vi "test2.vi"() -> ()   [LabVIEW 2023]
uses:
  Devices/Rigol DS1054/Rigol DS1054.lvclass
  D:/git/HAL/Scope Base/Scope Base.lvclass
  Camera Base/Acquisition Stats.ctl
  Devices/PXIe-5172 Simulated/PXIe-5172 Simulated.lvclass
  Devices/PXIe-5172 Simulated/configurations/Fetch 10kHz_class/Continuous Waveform Acq CFG.lvclass
  D:/git/HAL/Configuration Base/Configuration Base.lvclass
  Devices/Rigol DS1054/Configurations/Acquire Continuous Waveform/Continuous Waveform Acq CFG.lvclass
  Configuration Base/Configuration Base.lvclass
  D:/git/HAL/Interfaces/IConfigure/IConfigure.lvclass
  Scope Base/Scope Base.lvclass
  Devices/Flir A700/Flir A700.lvclass
  Camera Imaqdx/Configuration/Camera Imaqdx CFG.lvclass
  Camera Base/Camera Base.lvclass
  D:/git/HAL/Camera Base/Camera Base.lvclass
panel:
  out "Acquisition Stats":T1
  out "Image":T2(plugin-control)
  out "error out cams":errorcluster
  out "error out scopes":errorcluster
  out "Error Out":errorcluster
  in  "RIGOL DS1054.lvlib:Rigol DS1054.lvclass":refnum<class "Rigol DS1054.lvclass">
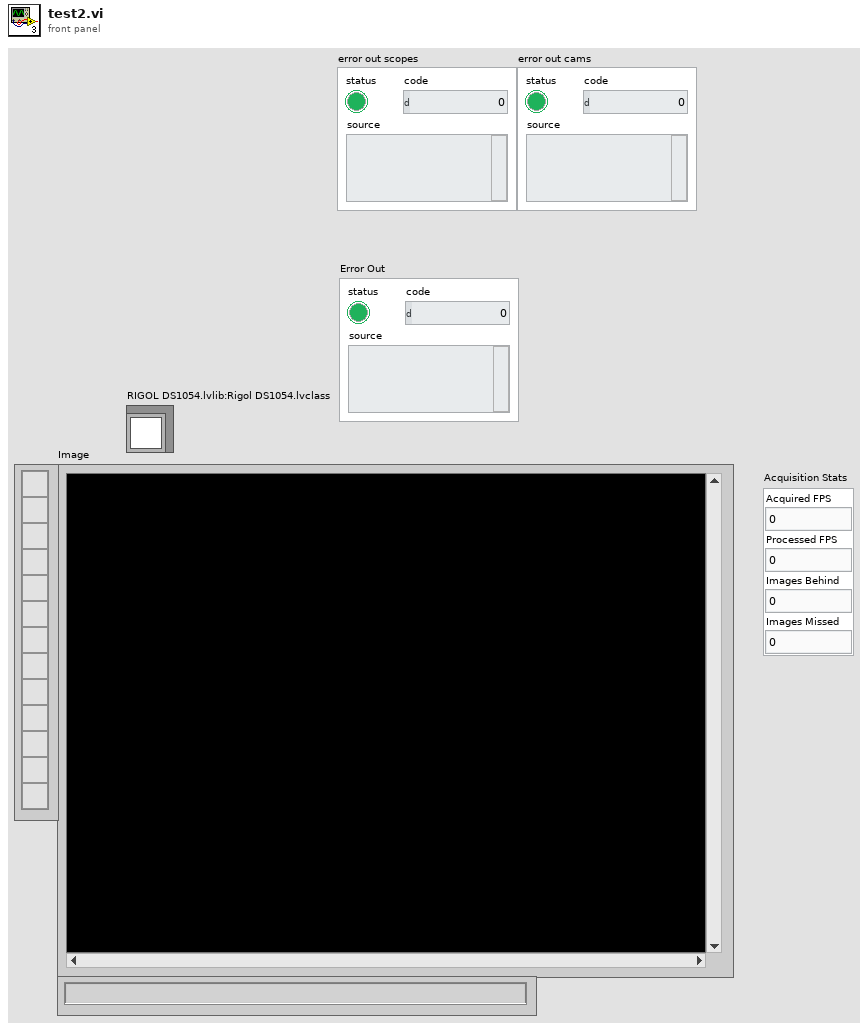
[diagram p1: front panel]
types:
  T1 = typedef "HAL.lvlib/Camera Base.lvclass/Acquisition Stats.ctl" = cluster{"Acquired FPS":dbl, "Processed FPS":dbl, "Images Behind":u32, "Images Missed":u32}
  T2 = typedef "IMAQ Image.ctl" = refnum<image>
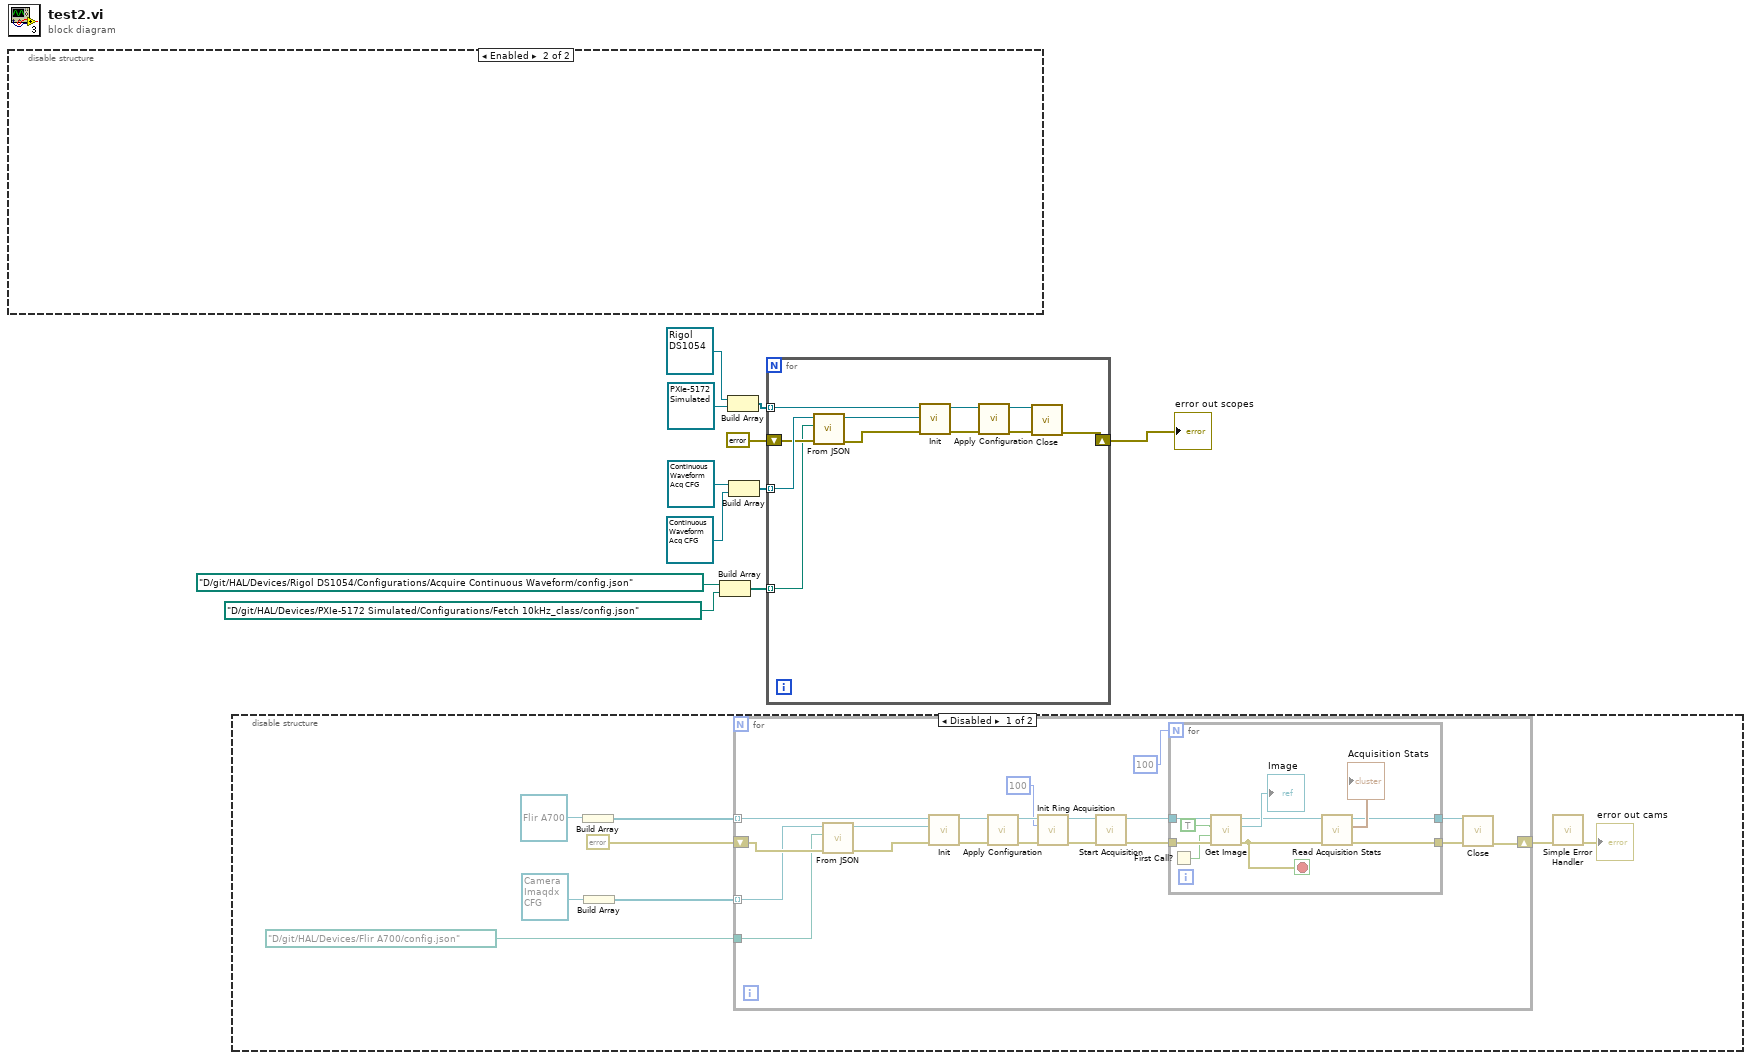
[diagram p0: block diagram]
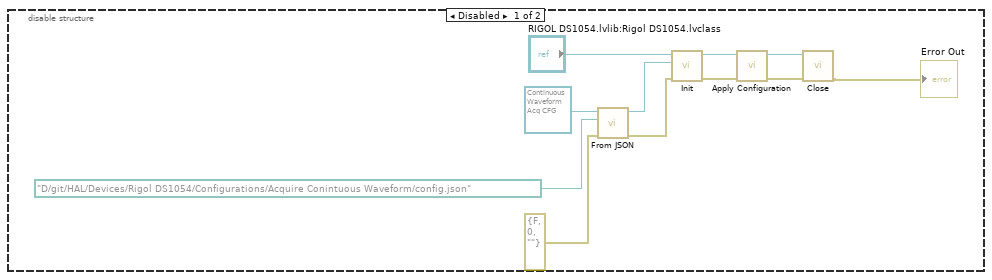
[diagram p3: hidden frame]
diagram:
  n1 = disable-structure shown="Enabled" {
    frame Disabled {
      n2 = call-dynamic "From JSON.vi"("error in (no error)"=errorcluster {"status"=FALSE, "code"=0, "source"=""} ("Error In"), "JSON Config"=path "D:/git/HAL/Devices/Rigol DS1054/Configurations/Acquire Conintuous Waveform/config.json" ("File Path"), "Camera Config in"=refnum<class "Continuous Waveform Acq CFG.lvclass"> refnum ("RIGOL DS1054.lvlib:Acquire Continuous Waveform CFG.lvclass")) -> ("error out"=w12:errorcluster, "Camera Config out"=w21:refnum<class "Continuous Waveform Acq CFG.lvclass">)  [unwired: 7 in]
      n3 = call-dynamic "Init.vi"("Error In"=w12, "IConfigure"=w21, "object in"="RIGOL DS1054.lvlib:Rigol DS1054.lvclass") -> ("Error Out"=w17:errorcluster, "object out"=w18:refnum<class "Rigol DS1054.lvclass">)  [unwired: 7 in]
      n4 = call "Apply Configuration.vi"("error in (no error)"=w17, "Rigol DS1054 in"=w18) -> ("error out"=w15:errorcluster, "Rigol DS1054 out"=w16:refnum<class "Rigol DS1054.lvclass">)  [unwired: 8 in]
      n5 = call-dynamic "Close.vi"("Error In"=w15, "object in"=w16) -> ("Error Out"=→"Error Out":errorcluster)  [unwired: 8 in, 1 out]
    }
    frame Enabled {
    }
  }
  n6 = disable-structure shown="Disabled" {
    frame Disabled {
      n7 = Build Array(refnum<class "Flir A700.lvclass"> refnum ("FLIR A700.lvlib:Flir A700.lvclass")) -> (w27:refnum<class "Flir A700.lvclass">[])
      n8 = Build Array(refnum<class "Camera Imaqdx CFG.lvclass"> refnum ("HAL.lvlib:Camera Imaqdx CFG.lvclass")) -> (w28:refnum<class "Camera Imaqdx CFG.lvclass">[])
      n9 = for {
        tunnel: w27 -> [w49] mode=indexing
        tunnel: w28 -> [w43] mode=indexing
        shift-right: [w45] -> w30
        shift-left: errorcluster {"status"=FALSE, "code"=0, "source"=""} ("error constant") -> [w48]
        tunnel: path "D:/git/HAL/Devices/Flir A700/config.json" ("JSON Config") -> [w41]
        n10 = call-dynamic "From JSON.vi"("error in"=w48, "JSON Config"=w41, "Camera Config Imaqdx in"=w43) -> ("error out"=w44:errorcluster, "Camera Config Imaqdx out"=w42:refnum<class "Camera Imaqdx CFG.lvclass">)  [unwired: 7 in]
        n11 = call-dynamic "Init.vi"("error in (no error)"=w44, "IConfigure"=w42, "Flir A700 in"=w49) -> ("error out"=w47:errorcluster, "Flir A700 out"=w46:refnum<class "Flir A700.lvclass">)  [unwired: 7 in]
        n12 = call-dynamic "Apply Configuration.vi"("error in (no error)"=w47, "Camera Base in"=w46) -> ("error out"=w39:errorcluster, "Camera Base out"=w38:refnum<class "Flir A700.lvclass">)  [unwired: 8 in]
        n13 = call-dynamic "Init Ring Acquisition.vi"("error in (no error)"=w39, "Ring Buffer Size"=u32 100, "Camera Imaqdx in"=w38) -> ("error out"=w36:errorcluster, "Camera Imaqdx out"=w35:refnum<class "Flir A700.lvclass">)  [unwired: 7 in]
        n14 = call-dynamic "Start Acquisition.vi"("error in"=w36, "Camera Imaqdx in"=w35) -> ("error out"=w33:errorcluster, "Camera Imaqdx out"=w34:refnum<class "Flir A700.lvclass">)  [unwired: 8 in]
        n15 = for {
          N: 100 -> [_]
          tunnel: w34 -> [w58]
          tunnel: w33 -> [w59]
          tunnel: [w51] -> w32
          tunnel: [w50] -> w31
          stop <- w54 stop-if-true
          n16 = First Call?() -> (First Call?: T/F=w55:bool)
          n17 = call-dynamic "Get Image.vi"("error in"=w59, "Reset Stats?"=w55, "Calc Stats?"=TRUE, "Camera Imaqdx in"=w58) -> ("error out"=w54:errorcluster, "Image out"=→"Image":T2, "Camera Imaqdx out"=w52:refnum<class "Flir A700.lvclass">)  [unwired: 5 in]
          n18 = call "Read Acquisition Stats.vi"("error in (no error)"=w54, "Camera Base in"=w52) -> ("error out"=w51:errorcluster, "Acquisition Stats"=→"Acquisition Stats":T1, "Camera Base out"=w50:refnum<class "Flir A700.lvclass">)  [unwired: 7 in]
        }
        n19 = call-dynamic "Close.vi"("error in (no error)"=w32, "Camera Base in"=w31) -> ("error out"=w45:errorcluster)  [unwired: 8 in, 1 out]
      }
      n20 = call <vilib>:"Simple Error Handler.vi"("error in (no error)"=w30) -> ("error out"=→"error out cams":errorcluster)  [unwired: 4 in, 4 out]
    }
    frame Enabled {
    }
  }
  n21 = Build Array(path "D:/git/HAL/Devices/Rigol DS1054/Configurations/Acquire Continuous Waveform/config.json" ("JSON Config"), path "D:/git/HAL/Devices/PXIe-5172 Simulated/Configurations/Fetch 10kHz_class/config.json" ("JSON Config")) -> (w2:path[])
  n22 = Build Array(refnum<class "Rigol DS1054.lvclass"> refnum ("RIGOL DS1054.lvlib:Rigol DS1054.lvclass"), refnum<class "PXIe-5172 Simulated.lvclass"> refnum ("PXIe-5172 Simulated.lvlib:PXIe-5172 Simulated")) -> (w10:refnum<class "Scope Base.lvclass">[])
  n23 = Build Array(refnum<class "Continuous Waveform Acq CFG.lvclass"> refnum ("RIGOL DS1054.lvlib:Continuous Waveform Acq CFG.lvclass"), refnum<class "Continuous Waveform Acq CFG.lvclass"> refnum ("PXIe-5172 Simulated.lvlib:Fetch 10kHz")) -> (w8:refnum<class "Configuration Base.lvclass">[])
  n24 = for {
    tunnel: w10 -> [w70] mode=indexing
    tunnel: w8 -> [w69] mode=indexing
    shift-right: [w64] -> w6
    shift-left: errorcluster {"status"=FALSE, "code"=0, "source"=""} ("error constant") -> [w62]
    tunnel: w2 -> [w60] mode=indexing
    n25 = call-dynamic "From JSON.vi"("error in (no error)"=w62, "JSON Config"=w60, "Camera Config in"=w69) -> ("error out"=w61:errorcluster, "Camera Config out"=w63:refnum<class "Configuration Base.lvclass">)  [unwired: 7 in]
    n26 = call-dynamic "Init.vi"("Error In"=w61, "HAL.lvlib:IConfigure"=w63, "object in"=w70) -> ("Error Out"=w68:errorcluster, "object out"=w67:refnum<class "Scope Base.lvclass">)  [unwired: 7 in]
    n27 = call-dynamic "Apply Configuration.vi"("error in"=w68, "Scope Base in"=w67) -> ("error out"=w65:errorcluster, "Scope Base out"=w66:refnum<class "Scope Base.lvclass">)  [unwired: 8 in]
    n28 = call-dynamic "Close.vi"("Error In"=w65, "object in"=w66) -> ("Error Out"=w64:errorcluster)  [unwired: 8 in, 1 out]
  }
  "error out scopes" <- w6
